vi "Write Q0 params.vi"(8 "error in (no error)":errorcluster, 10 "Q0 params":T1, 11 "Scope5761 in":refnum<class "Scope5782_six_channel.lvclass">) -> (0 "error out":errorcluster, 3 "Scope5761out":refnum<class "Scope5782_six_channel.lvclass">)   [LabVIEW 2018, in "Scope5782_six_channel.lvclass"]
uses:
  Scope5782_six_channel.lvclass
  Q0 params.ctl
  Scope5782_six_channel.lvclass/Scope5782_six_channel.ctl
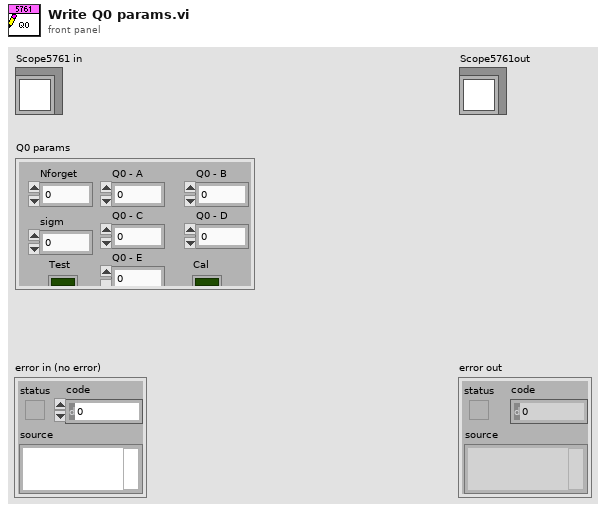
[diagram p1: front panel]
types:
  T1 = typedef "Scope5782_six_channel.lvclass/Q0 params.ctl" = cluster{"Nforget":i32, "sigm":dbl, "Q0 - A":dbl, "Q0 - B":dbl, "Q0 - C":dbl, "Q0 - D":dbl, "Q0 - E":dbl, "Test":bool, "Cal":bool}
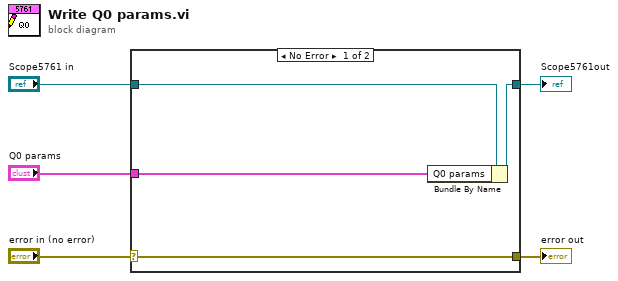
[diagram p0: block diagram]
diagram:
  n1 = case shown="No Error" "error in (no error)" {
    selector: "error in (no error)" -> [w9 w10]
    tunnel: [w9 w10] -> w4
    tunnel: [w7 w11] -> w2
    tunnel: "Scope5761 in" -> [w8 w11]
    tunnel: "Q0 params" -> [w6 _]
    frame No Error {
      n2 = Bundle By Name(cluster=w8, "Q0 params"=w6) -> (w7:refnum<class "Scope5782_six_channel.lvclass">)
    }
    frame Error {
    }
  }
  "error out" <- w4
  "Scope5761out" <- w2
